vi "Configure Save On Event.vi"(0 "VISA resource name":refnum<visa-resource-name>, 5 "Enable Save On Event (F:Disable)":bool, 7 "Events Type (0:Limit Evaluation Fail)":i32(ring) items=["Limit Evaluation Fail", "Limit Evaluation Pass", "Margin Evaluation Fail", "Margin Evaluation Pass", "Sweep"], 9 "Enable Save Then Stop (F:Disable)":bool, 11 "error in (no error)":errorcluster) -> (4 "VISA resource name out":refnum<visa-resource-name>, 15 "error out":errorcluster)   [LabVIEW 2020, in "Anritsu Signal Analyzer Series.lvlib"]
doc: "Configures the save on event settings of the spectrum analyzer."
uses:
  Anritsu Signal Analyzer Series.lvlib
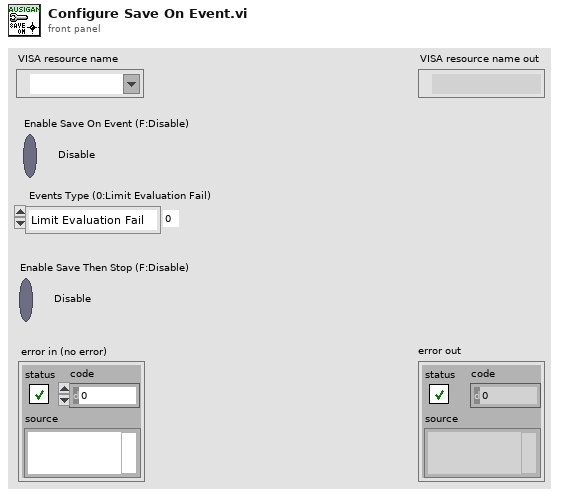
[diagram p1: front panel]
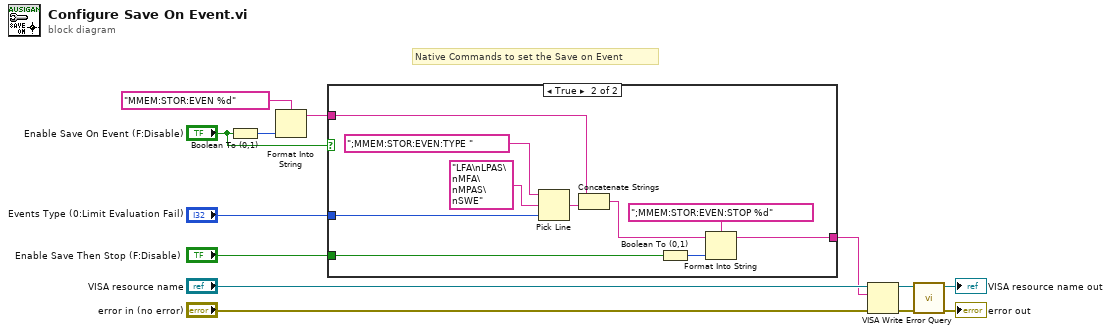
[diagram p0: block diagram]
diagram:
  # "Native Commands to set the Save on Event"
  n1 = Boolean To (0,1)(Boolean="Enable Save On Event (F:Disable)") -> (0, 1=w5:i16)
  n2 = Format Into String(format string="MMEM:STOR:EVEN %d" ("Format String"), w5) -> (resulting string=w1:string)  [unwired: 2 in, 1 out]
  n3 = case shown="True" "Enable Save On Event (F:Disable)" {
    tunnel: "Events Type (0:Limit Evaluation Fail)" -> [_ w23]
    tunnel: "Enable Save Then Stop (F:Disable)" -> [_ w21]
    tunnel: [w14 w18] -> w3
    tunnel: w1 -> [w14 w17]
    frame False {
    }
    frame True {
      n4 = Pick Line(string ("")=";MMEM:STOR:EVEN:TYPE ", multi-line string="LFA\nLPAS\nMFA\nMPAS\nSWE", line index=w23) -> (output string=w16:string)
      n5 = Concatenate Strings(w17, w16) -> (w15:string)
      n6 = Boolean To (0,1)(Boolean=w21) -> (0, 1=w20:i16)
      n7 = Format Into String(format string=";MMEM:STOR:EVEN:STOP %d" ("Format String"), initial string=w15, w20) -> (resulting string=w18:string)  [unwired: 1 in, 1 out]
    }
  }
  n8 = VISA Write(VISA resource name="VISA resource name", write buffer=w3, error in (no error)="error in (no error)") -> (VISA resource name out=w9:refnum<visa-resource-name>, error out=w10:errorcluster)  [unwired: 1 out]
  n9 = call "Error Query.vi"("error in (no error)"=w10, "VISA resource name"=w9) -> ("error out"=→"error out":errorcluster, "VISA resource name out"=→"VISA resource name out":refnum<visa-resource-name>)  [unwired: 6 in, 2 out]
